vi "Write Default to File.vi"(8 "error in (no error)":errorcluster, 9 "Name":string, 10 "Path":path, 11 "Dot Settings in":refnum<class "Dot Settings.lvclass">) -> (0 "error out":errorcluster, 3 "Dot Settings out":refnum<class "Dot Settings.lvclass">)   [LabVIEW 2019, in "Dot Settings.lvclass"]
uses:
  Dot Settings.lvclass
  ObjectSettings/ObjectSettings.lvclass
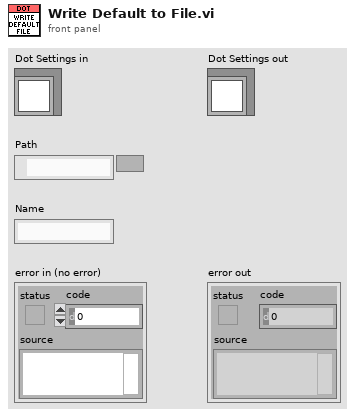
[diagram p1: front panel]
types:
  T1 = typedef "Dot Settings.lvclass/Default Dot Cluster.ctl" = cluster{"Action":T2, "Dot KVPs":cluster{"Key":string, "Value":string}[]}
  T2 = typedef "Dot Settings.lvclass/Action.ctl" = enum16{"IV", "QD"}
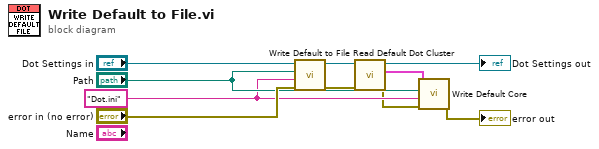
[diagram p0: block diagram]
diagram:
  w3 = "Dot.ini" ("Name")
  n1 = call-parent "Write Default to File.vi"("error in (no error)"="error in (no error)", "Name"=w3, "Path"="Path", "ObjectSettings in"="Dot Settings in") -> ("error out"=w6:errorcluster, "ObjectSettings out"=w8:refnum<class "Dot Settings.lvclass">)  [unwired: 6 in]
  n2 = call "Read Default Dot Cluster.vi"("error in (no error)"=w6, "Dot Settings in"=w8) -> ("error out"=w2:errorcluster, "Default Dot"=w5:T1, "Dot Settings out"=→"Dot Settings out":refnum<class "Dot Settings.lvclass">)  [unwired: 7 in]
  n3 = call "Write Default Core.vi"("error in (no error)"=w2, "Name"=w3, "Path"="Path", "Cluster In"=w5) -> ("error out"=→"error out":errorcluster)  [unwired: 6 in, 1 out]
